vi "sub vi - AI USB4704 (3)  Close Task v1.vi"(0 "TASK USB 0":i32, 5 "TASK USB 1":i32, 7 "TASK USB 2":i32) -> ()   [LabVIEW 2013]
panel:
  out "error array":errorcluster[](array[cluster])
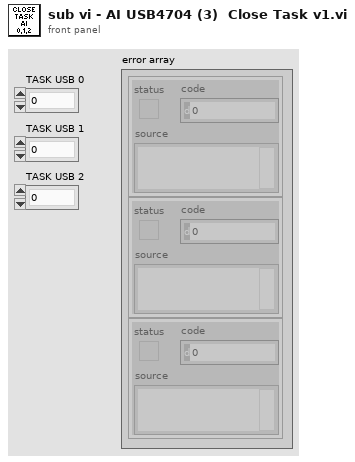
[diagram p1: front panel]
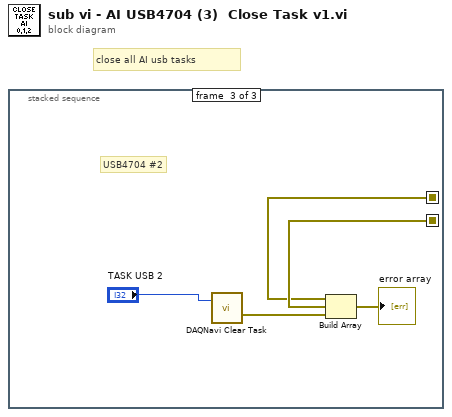
[diagram p0: block diagram]
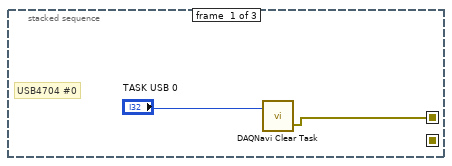
[diagram p2: hidden frame]
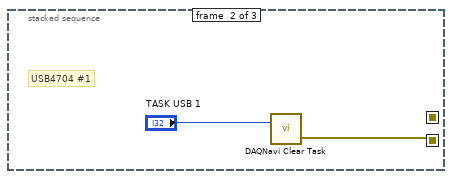
[diagram p3: hidden frame]
diagram:
  # "close all AI usb tasks"
  n1 = stacked-sequence {
    seq-local: [w2 _ _] -> [_ _ w7]
    seq-local: [_ w4 _] -> [_ _ w8]
    frame #0 {
      # "USB4704 #0"
      n2 = call <userlib>:"DAQNavi Clear Task.vi"("task in"="TASK USB 0") -> ("error out"=w2:errorcluster)  [unwired: 1 in, 1 out]
    }
    frame #1 {
      # "USB4704 #1"
      n3 = call <userlib>:"DAQNavi Clear Task.vi"("task in"="TASK USB 1") -> ("error out"=w4:errorcluster)  [unwired: 1 in, 1 out]
    }
    frame #2 {
      # "USB4704 #2"
      n4 = call <userlib>:"DAQNavi Clear Task.vi"("task in"="TASK USB 2") -> ("error out"=w9:errorcluster)  [unwired: 1 in, 1 out]
      n5 = Build Array(w7, w8, w9) -> (→"error array":errorcluster[])
    }
  }
